vi "Panel-OED.vi"() -> ()   [LabVIEW 2009]
uses:
  Instruments/Motor/Controls/MotorStatus.ctl
panel:
  out "OED2-POL":T1
  out "OED1-POL":T1
  out "OED2-FI-X":T1
  out "OED2-FI-Y":T1
  out "OED2-FI-Z":T1
  in  "stop":bool
  out "OED1-FI-Z":T1
  out "OED1-FI-Y":T1
  out "OED1-FI-X":T1
  # "OED1-FI"
  # "OED2-FI"
  # "POL1"
  # "POL2"
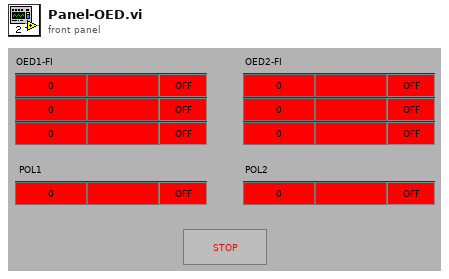
[diagram p1: front panel]
types:
  T1 = typedef "MotorStatus.ctl" = cluster{"Managed?":bool, "Position":i32, "Name":string, "Status":enum16{"OFF", "IDLE", "MOVING", "HOMING"}}
  T2 = enum32{"Invalid", "Standard", "Closed", "Hidden", "Minimized", "Maximized"}
  T3 = enum32{"Bad", "Idle", "Run top level", "Running"}
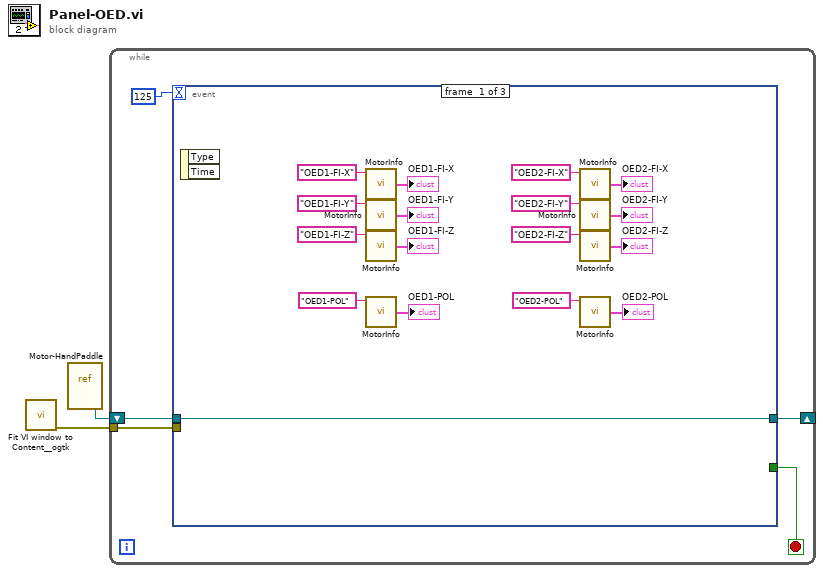
[diagram p0: block diagram]
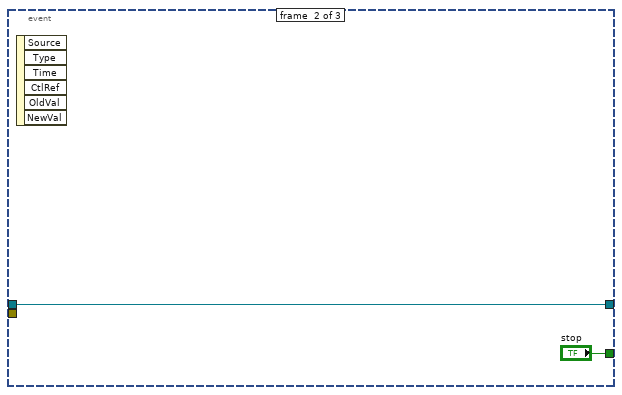
[diagram p2: hidden frame]
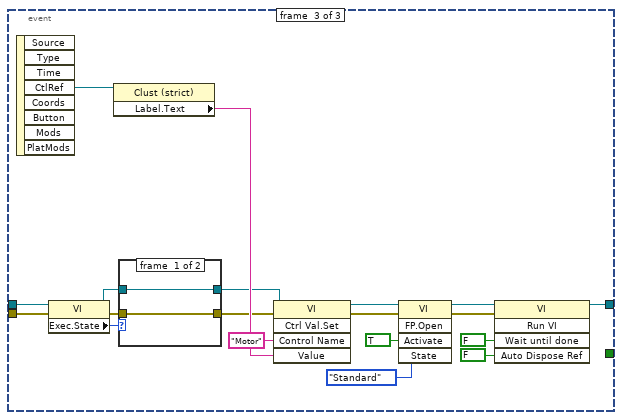
[diagram p3: hidden frame]
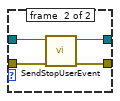
[diagram p4: hidden frame]
diagram:
  n1 = call <userlib>:"Fit VI window to Content__ogtk.vi"() -> ("error out"=w1:errorcluster)  [unwired: 3 in, 4 out]
  n2 = vi-ref "Motor-HandPaddle.vi"() -> (w2:refnum<vi>)
  n3 = while {
    shift-right: [w6] -> _
    shift-left: w2 -> [w5]
    tunnel: w1 -> [w3]
    stop <- w4 stop-if-true
    n4 = event shown="[2] \"OED1-FI-X\", \"OED1-FI-Y\", \"OED1-FI-Z\", \"OED2-FI-Z\", \"OED2-FI-X\", \"OED2-FI-Y\", \"OED1-POL\", \"OED2-POL\": Mouse Down" {
      selector: _ -> [_ _ _]
      dyn-events: _ -> [_ _ _]
      timeout: 125 -> [_ _ _]
      tunnel: [_ "stop" _] -> w4
      tunnel: [w12 w25 w35] -> w6
      tunnel: w5 -> [w12 w25 w33]
      tunnel: w3 -> [_ _ w27]
      event #0 {
        n5 = event-data() -> ()  [unwired: 3 out]
        n6 = call "MotorInfo.vi"("Motor"="OED1-FI-X") -> ("Axis status"=→"OED1-FI-X":T1)  [unwired: 1 in, 7 out]
        n7 = call "MotorInfo.vi"("Motor"="OED1-FI-Y") -> ("Axis status"=→"OED1-FI-Y":T1)  [unwired: 1 in, 7 out]
        n8 = call "MotorInfo.vi"("Motor"="OED1-FI-Z") -> ("Axis status"=→"OED1-FI-Z":T1)  [unwired: 1 in, 7 out]
        n9 = call "MotorInfo.vi"("Motor"="OED1-POL") -> ("Axis status"=→"OED1-POL":T1)  [unwired: 1 in, 7 out]
        n10 = call "MotorInfo.vi"("Motor"="OED2-FI-X") -> ("Axis status"=→"OED2-FI-X":T1)  [unwired: 1 in, 7 out]
        n11 = call "MotorInfo.vi"("Motor"="OED2-FI-Y") -> ("Axis status"=→"OED2-FI-Y":T1)  [unwired: 1 in, 7 out]
        n12 = call "MotorInfo.vi"("Motor"="OED2-FI-Z") -> ("Axis status"=→"OED2-FI-Z":T1)  [unwired: 1 in, 7 out]
        n13 = call "MotorInfo.vi"("Motor"="OED2-POL") -> ("Axis status"=→"OED2-POL":T1)  [unwired: 1 in, 7 out]
      }
      event #1 {
        n14 = event-data() -> ()  [unwired: 7 out]
      }
      event #2 {
        n15 = event-data() -> ("CtlRef"=w45:refnum<vi>)  [unwired: 8 out]
        n16 = property class="VI"(reference=w33, error in=w27) -> (reference out=w29:refnum<vi>, error out=w30:errorcluster, "Exec.State"=w32:T3)
        n17 = property class="Clust (strict)"(reference=w45) -> ("Label.Text"=w34:string)  [unwired: 1 in, 2 out]
        n18 = case shown="\"Run top level\", \"Running\"" w32 {
          tunnel: w29 -> [w47 w51]
          tunnel: [w47 w48] -> w28
          tunnel: [w46 w49] -> w31
          tunnel: w30 -> [w46 w50]
          frame #0 {
          }
          frame #1 {
            n19 = call "SendStopUserEvent.vi"("VI Refnum in"=w51, "error in"=w50) -> ("VI Refnum out"=w48:refnum<vi>, "error out"=w49:errorcluster)  [unwired: 6 out]
          }
        }
        n20 = invoke class="VI" method="Ctrl Val.Set"(reference=w28, error in=w31, "Control Name"="Motor", "Value"=w34) -> (reference out=w36:refnum<vi>, error out=w41:errorcluster)  [unwired: 1 in, 3 out]
        n21 = invoke class="VI" method="FP.Open"(reference=w36, error in=w41, "Activate"=TRUE ("Activate?"), "State"=T2."Standard") -> (reference out=w39:refnum<vi>, error out=w40:errorcluster)  [unwired: 1 in, 3 out]
        n22 = invoke class="VI" method="Run VI"(reference=w39, error in=w40, "Wait until done"=FALSE ("Wait Until Done"), "Auto Dispose Ref"=FALSE ("Auto Dispose Reference")) -> (reference out=w35:refnum<vi>)  [unwired: 1 in, 4 out]
      }
    }
  }
